vi "CCD ShutterSetup0.1.vi"(2 "Shutter Enabled":bool=TRUE, 3 "Exposure time":dbl=0.2 format="%.2f") -> (0 "ExpTime string":string="ex0.20", 1 "ExpTime returned":dbl=0.2 format="%.2f")   [LabVIEW 2019]
doc: "Sets the exposure time and shutter action for the \nnext CCD shot. Exposure time is returned between \n0.02 and 6000s. This VI uses the Global variable \nCCDsetupGLOBAL.var for CCD GPIB address and \nexposure-time and -string as well as shutter action."
uses:
  Globals and TypeDefs/CCDsetupGLOBAL.vi
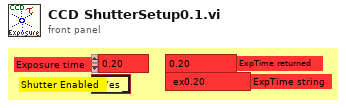
[diagram p1: front panel]
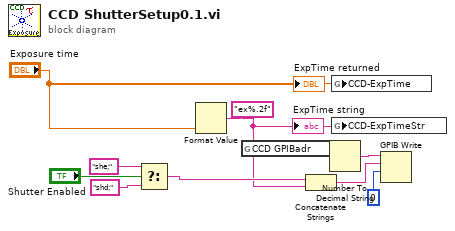
[diagram p0: block diagram]
diagram:
  n1 = Select(t="she;", s="Shutter Enabled", f="shd;") -> (s? t:f=w10:string)
  n2 = Format Value(format string="ex%.2f", value (0)="Exposure time") -> (output string=w6:string)  [unwired: 1 in]
  "ExpTime string" <- w6
  n3 = global read "CCDsetupGLOBAL.vi" "CCD GPIBadr"() -> (w5:i16)
  n4 = Concatenate Strings(w10, w6) -> (w3:string)
  n5 = Number To Decimal String(number=w5) -> (decimal integer string=w4:string)  [unwired: 1 in]
  n6 = global write "CCDsetupGLOBAL.vi" "CCD-ExpTime"("Exposure time") -> ()
  n7 = global write "CCDsetupGLOBAL.vi" "CCD-ExpTimeStr"(w6) -> ()
  n8 = GPIB Write(0:w4, 1:w3, 2:u8 0) -> ()  [unwired: 2 in, 2 out]
  "ExpTime returned" <- "Exposure time"
